vi "HorseChase.vi"() -> ()   [LabVIEW 2018]
uses:
  <vilib>/Rock Robotics/WPI/ThirdParty/Phoenix-LabVIEW/Motor Controller/Controls/CTRE_Phoenix_MotorControl_ControlMode.ctl
  <vilib>/Rock Robotics/WPI/ThirdParty/Phoenix-LabVIEW/Motor Controller/Get/CTRE_Phoenix_MotorController_GetSelectedSensorData.vi
  <vilib>/addons/control/pid/pid.llb/PID (DBL).vi
  <vilib>/addons/control/pid/NI_PID_pid.lvlib
panel:
  out "Position (Raw Sensor Units)":i32
  in  "Horse Toggle":bool
  in  "Negative":bool
  in  "Positive":bool
  in  "Boolean 7":bool
  in  "Boolean 6":bool
  in  "Numeric 2":dbl format="%#_13g"
  in  "Numeric":dbl format="%#_13g"
  in  "Boolean 5":bool
  in  "Boolean 3":bool
  in  "Boolean 4":bool
  in  "Boolean 2":bool
  in  "Boolean":bool
  in  "Max Encoder Posistion":dbl format="%#_13g"
  in  "Joystick Information":dbl format="%#_13g"
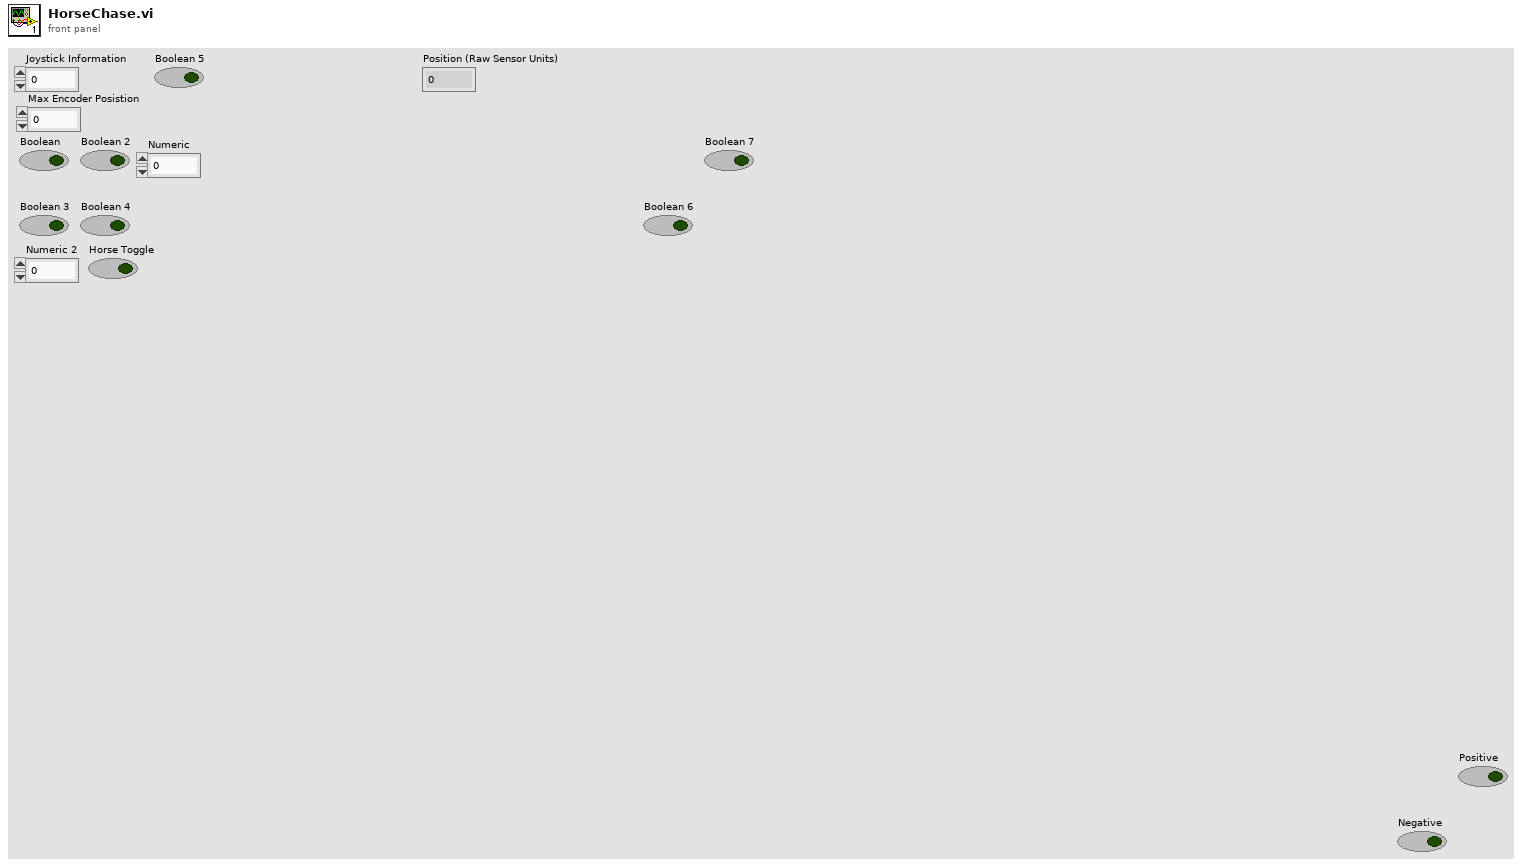
[diagram p1: front panel]
types:
  T1 = typedef "CTRE_Phoenix_MotorControl_ControlMode.ctl" = u16
  T2 = enum16{"Resting", "CargoShip Front", "CargoShip Back", "Cargo Mid", "Hatch Mid", "All High", "Cargo Intake"}
  T3 = enum16{"Resting", "Hatch Ground Intake", "Hatch Place Low/Mid/CargoShip", "Hatch Place High", "Cargo Ground Intake", "Cargo Place Low/Mid", "Cargo Place High", "CargoShip Place Front", "CargoShip Place Back"}
  T4 = cluster{"proportional gain (Kc)":dbl, "integral time (Ti, min)":dbl, "derivative time (Td, min)":dbl}
  T5 = typedef "WPI_MotorControlDeviceRef.ctl" = cluster{"DeviceStatus":errorcluster, "Type":T6, "PWM":cluster{"PWM Channel":T7, "DeadBand":T8}, "CAN":cluster{"Device Number":u8, "SetOutput VI Ref":variant, "GetOutput VI Ref":variant, "Enable VI Ref":variant, "Disable VI Ref":variant, "Data":variant}, "Invert":bool, "DIO PWM":cluster{"PWM \"Enable\" Channel":T7, "DIOChannel":T9, "PWM Rate":dbl}}
  T6 = typedef "WPI_MotorControlType.ctl" = enum16{"PWM", "CAN", "DIO PWM"}
  T7 = typedef "FPGA_DIOPWMChannel.ctl" = enum8{"PWM 0", "PWM 1", "PWM 2", "PWM 3", "PWM 4", "PWM 5", "PWM 6", "PWM 7", "PWM 8", "PWM 9", "PWM MXP 0", "PWM MXP 1", "PWM MXP 2", "PWM MXP 3", "PWM MXP 4", "PWM MXP 5", "PWM MXP 6", "PWM MXP 7", "PWM MXP 8", "PWM MXP 9", "Invalid"}
  T8 = typedef "WPI_PWMDeadband.ctl" = cluster{"Name":string, "maxPositivePwm":i32, "minPositivePwm":i32, "centerPwm":i32, "maxNegativePwm":i32, "minNegativePwm":i32, "angularRange":u16}
  T9 = typedef "FPGA_DIOChannel.ctl" = enum8{"DIO 0", "DIO 1", "DIO 2", "DIO 3", "DIO 4", "DIO 5", "DIO 6", "DIO 7", "DIO 8", "DIO 9", "DIO MXP 0", "DIO MXP 1", "DIO MXP 2", "DIO MXP 3", "DIO MXP 4", "DIO MXP 5", "DIO MXP 6", "DIO MXP 7", "DIO MXP 8", "DIO MXP 9", "DIO MXP 10", "DIO MXP 11", "DIO MXP 12", "DIO MXP 13", "DIO MXP 14", "DIO MXP 15", "SPI Port CS1", "SPI Port CS2", "SPI Port CS3", "SPI Port MISO", "SPI Port MOSI", "Invalid"}
  T10 = typedef "WPI_SwitchDevRef.ctl" = cluster{"DevStatus":errorcluster, "DIO Channel":T9, "CntIndex":T11, "Normally Closed":bool}
  T11 = typedef "FPGA_CounterCtrSystemIndex.ctl" = enum8{"Ctr 0", "Ctr 1", "Ctr 2", "Ctr 3", "Ctr 4", "Ctr 5", "Ctr 6", "Ctr 7", "Invalid"}
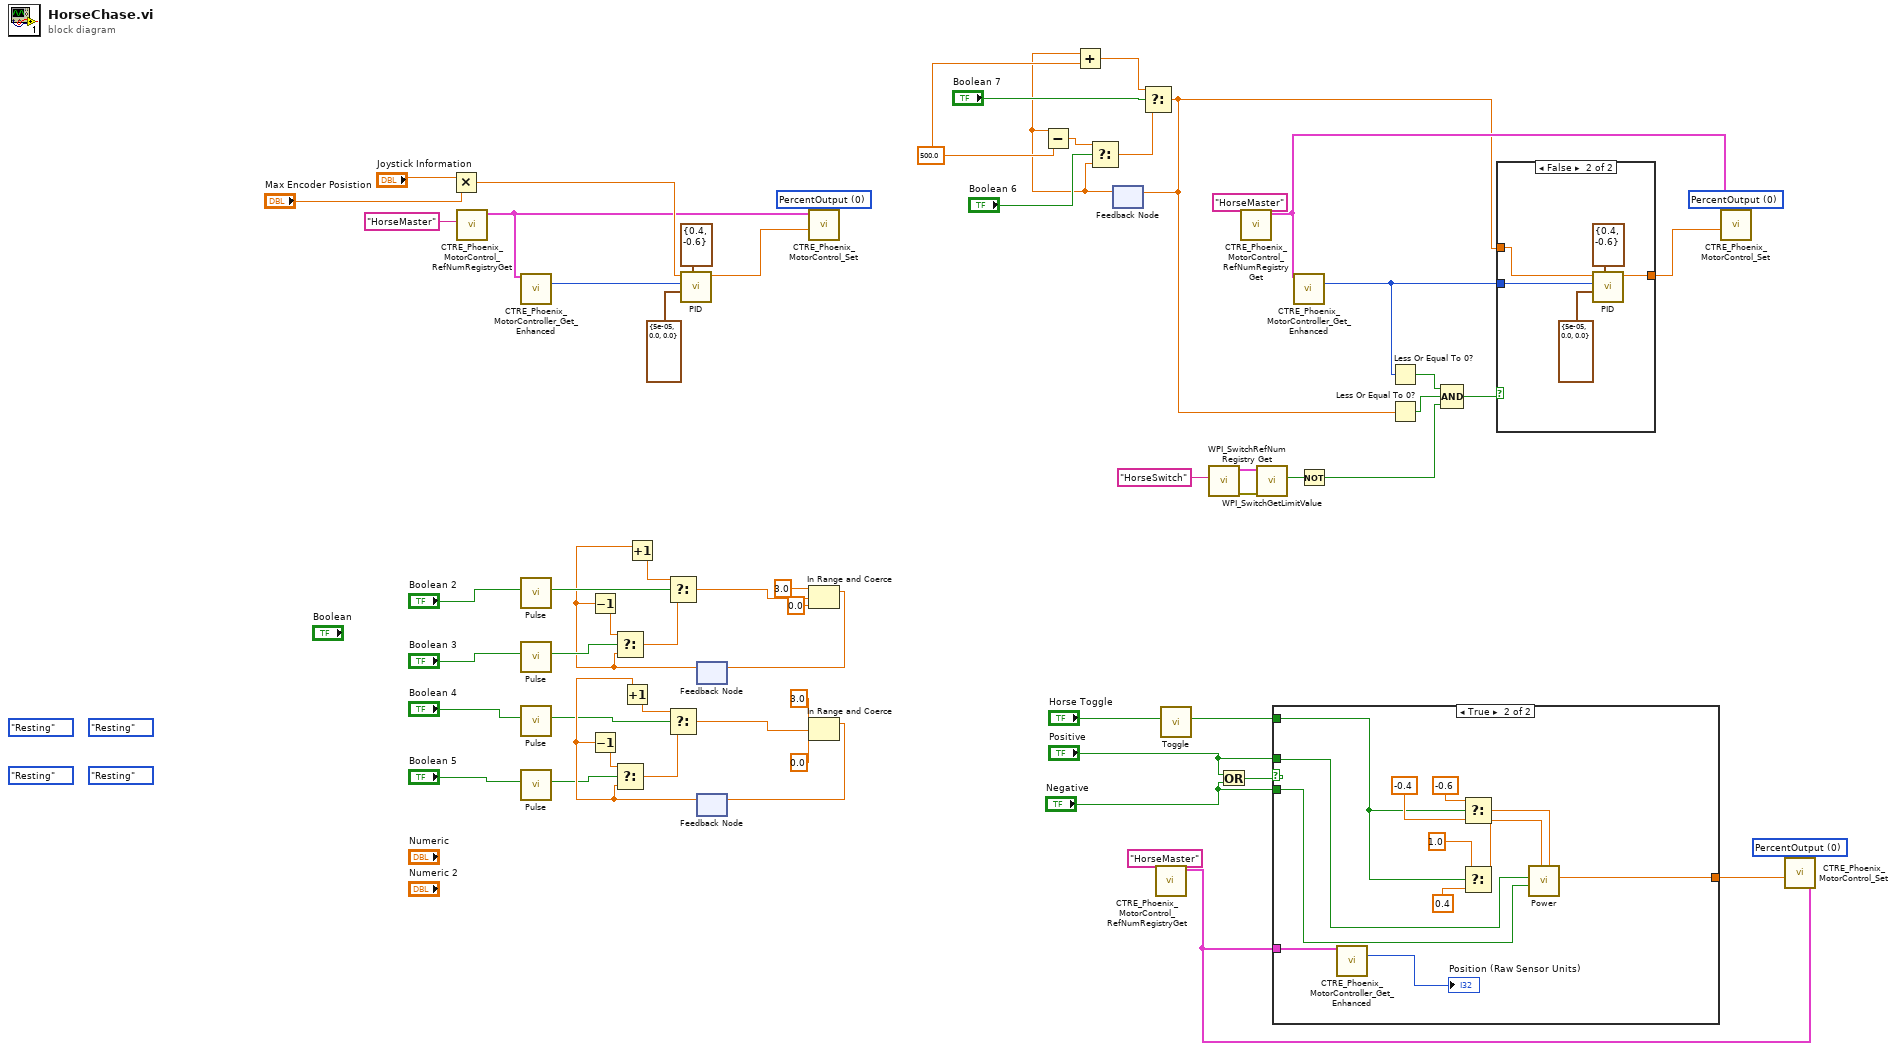
[diagram p0: block diagram]
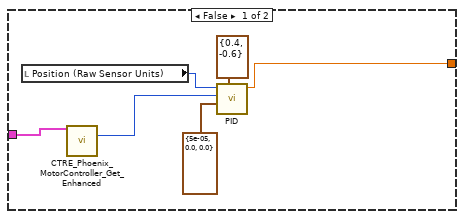
[diagram p2: hidden frame]
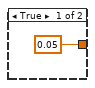
[diagram p3: hidden frame]
diagram:
  w5 = T1 0 items=["PercentOutput"=0, "Position"=1, "Velocity"=2, "Current"=3, "Follower"=5, "MotionProfile"=6, "MotionMagic"=7, "MotionProfileArc"=10, "Disabled"=15] ("Control Mode")
  (unwired) "HorseMaster" ("refnum name")
  w20 = 500.0 ("y")
  w29 = T1 0 items=["PercentOutput"=0, "Position"=1, "Velocity"=2, "Current"=3, "Follower"=5, "MotionProfile"=6, "MotionMagic"=7, "MotionProfileArc"=10, "Disabled"=15] ("Control Mode")
  (unwired) T2."Resting" ("Elevator Level Select")
  (unwired) T2."Resting" ("Elevator Level Select")
  (unwired) T3."Resting" ("Wrist")
  (unwired) T3."Resting" ("Wrist")
  w54 = T1 0 items=["PercentOutput"=0, "Position"=1, "Velocity"=2, "Current"=3, "Follower"=5, "MotionProfile"=6, "MotionMagic"=7, "MotionProfileArc"=10, "Disabled"=15] ("Control Mode")
  n1 = Multiply(x="Joystick Information", y="Max Encoder Posistion") -> (x*y=w60:dbl)
  n2 = call <vilib>:"CTRE_Phoenix_MotorControl_RefNumRegistryGet.vi"("refnum name"="HorseMaster") -> ("PhoenixMotorControlDevRef"=w55:T5)  [unwired: 9 in, 1 out]
  n3 = call-poly <vilib>:"CTRE_Phoenix_MotorController_Get_Enhanced.vi"("PhoenixMotorControlDevRef"=w55) -> ("Position (Raw Sensor Units)"=w59:i32)  [unwired: 11 in, 3 out]
  n4 = call "Pulse.vi"("Input"="Boolean 2") -> ("Output"=w52:bool)  [unwired: 10 in]
  n5 = call "Pulse.vi"("Input"="Boolean 3") -> ("Output"=w45:bool)  [unwired: 10 in]
  n6 = call "Pulse.vi"("Input"="Boolean 4") -> ("Output"=w32:bool)  [unwired: 10 in]
  n7 = call "Pulse.vi"("Input"="Boolean 5") -> ("Output"=w38:bool)  [unwired: 10 in]
  n8 = call-poly <vilib>:"PID.vi"("output range"=cluster{"output high":dbl, "output low":dbl} {"output high"=0.4, "output low"=-0.6}, "PID gains"=T4 {"proportional gain (Kc)"=5e-05, "integral time (Ti, min)"=0.0, "derivative time (Td, min)"=0.0}, "process variable"=w59, "setpoint"=w60) -> ("output"=w56:dbl)  [unwired: 6 in, 1 out]
  n9 = feedback #1() -> (w42:dbl)  [unwired: 1 in]
  n10 = Decrement(x=w42) -> (x-1=w43:dbl)
  n11 = Select(t=w43, s=w45, f=w42) -> (s? t:f=w46:dbl)
  n12 = Increment(x=w42) -> (x+1=w51:dbl)
  n13 = Select(t=w51, s=w52, f=w46) -> (s? t:f=w50:dbl)
  n14 = feedback #2() -> (w41:dbl)  [unwired: 1 in]
  n15 = Decrement(x=w41) -> (x-1=w40:dbl)
  n16 = Select(t=w40, s=w38, f=w41) -> (s? t:f=w37:dbl)
  n17 = Increment(x=w41) -> (x+1=w33:dbl)
  n18 = Select(t=w33, s=w32, f=w37) -> (s? t:f=w34:dbl)
  n19 = call <vilib>:"CTRE_Phoenix_MotorControl_Set.vi"("Output"=w56, "Control Mode"=w54, "PhoenixMotorControlDevRef"=w55) -> ()  [unwired: 7 in, 2 out]
  n20 = In Range and Coerce(upper limit=3.0, x=w50, lower limit=0.0) -> (coerced(x)=w44:dbl)  [unwired: 1 out]
  n21 = feedback-in #1(w44) -> ()
  n22 = In Range and Coerce(upper limit=3.0, x=w34, lower limit=0.0) -> (coerced(x)=w39:dbl)  [unwired: 1 out]
  n23 = feedback-in #2(w39) -> ()
  n24 = feedback #3() -> (w19:dbl)  [unwired: 1 in]
  n25 = Subtract(x=w19, y=w20) -> (x-y=w21:dbl)
  n26 = Add(x=w19, y=w20) -> (x+y=w22:dbl)
  n27 = Select(t=w21, s="Boolean 6", f=w19) -> (s? t:f=w25:dbl)
  n28 = Select(t=w22, s="Boolean 7", f=w25) -> (s? t:f=w18:dbl)
  n29 = feedback-in #3(w18) -> ()
  n30 = call <vilib>:"CTRE_Phoenix_MotorControl_RefNumRegistryGet.vi"() -> ("PhoenixMotorControlDevRef"=w4:T5)  [unwired: 10 in, 1 out]
  n31 = call "Toggle.vi"("Input"="Horse Toggle") -> ("Output"=w2:bool)  [unwired: 10 in]
  n32 = call <vilib>:"WPI_SwitchRefNum Registry Get.vi"("refnum name"="HorseSwitch") -> ("error out"=w14:errorcluster, "SwitchDevRef"=w13:T10)  [unwired: 9 in]
  n33 = Or(x="Positive", y="Negative") -> (x .or. y?=w8:bool)
  n34 = call <vilib>:"CTRE_Phoenix_MotorControl_RefNumRegistryGet.vi"("refnum name"="HorseMaster") -> ("PhoenixMotorControlDevRef"=w28:T5)  [unwired: 9 in, 1 out]
  n35 = call <vilib>:"WPI_SwitchGetLimitValue.vi"("error in (no error)"=w14, "SwitchDevRef"=w13) -> ("Switch Pressed"=w11:bool)  [unwired: 7 in, 2 out]
  n36 = case shown="True" w8 {
    tunnel: "Positive" -> [_ w75]
    tunnel: "Negative" -> [_ w74]
    tunnel: [w64 w73] -> w3
    tunnel: w4 -> [w69 w72]
    tunnel: w2 -> [_ w70]
    frame False {
      n37 = local read "Position (Raw Sensor Units)"() -> (w65:i32)
      n38 = call-poly <vilib>:"CTRE_Phoenix_MotorController_Get_Enhanced.vi"("PhoenixMotorControlDevRef"=w69) -> ("Position (Raw Sensor Units)"=w66:i32)  [unwired: 11 in, 3 out]
      n39 = call-poly <vilib>:"PID.vi"("output range"=cluster{"output high":dbl, "output low":dbl} {"output high"=0.4, "output low"=-0.6}, "PID gains"=T4 {"proportional gain (Kc)"=5e-05, "integral time (Ti, min)"=0.0, "derivative time (Td, min)"=0.0}, "process variable"=w66, "setpoint"=w65) -> ("output"=w64:dbl)  [unwired: 6 in, 1 out]
    }
    frame True {
      n40 = call-poly <vilib>:"CTRE_Phoenix_MotorController_Get_Enhanced.vi"("PhoenixMotorControlDevRef"=w72) -> ("Position (Raw Sensor Units)"=→"Position (Raw Sensor Units)":i32)  [unwired: 11 in, 3 out]
      n41 = Select(t=-0.6 ("f"), s=w70, f=-0.4) -> (s? t:f=w79:dbl)
      n42 = Select(t=1.0 ("f"), s=w70, f=0.4) -> (s? t:f=w78:dbl)
      n43 = call "Power.vi"("Negative Power"=w79, "Positive Power"=w78, "Negative"=w74, "Positive"=w75) -> ("Output"=w73:dbl)  [unwired: 7 in]
    }
  }
  n44 = call-poly <vilib>:"CTRE_Phoenix_MotorController_Get_Enhanced.vi"("PhoenixMotorControlDevRef"=w28) -> ("Position (Raw Sensor Units)"=w17:i32)  [unwired: 11 in, 3 out]
  n45 = Not(x=w11) -> (.not. x?=w10:bool)
  n46 = Less Or Equal To 0?(x=w17) -> (x <= 0?=w16:bool)
  n47 = Less Or Equal To 0?(x=w18) -> (x <= 0?=w15:bool)
  n48 = Compound Arithmetic op=AND(w16, w15, w10) -> (w9:bool)
  n49 = case shown="False" w9 {
    tunnel: [0.05 ("output") w87] -> w27
    tunnel: w17 -> [_ w84]
    tunnel: w18 -> [_ w83]
    frame True {
    }
    frame False {
      n50 = call-poly <vilib>:"PID.vi"("output range"=cluster{"output high":dbl, "output low":dbl} {"output high"=0.4, "output low"=-0.6}, "PID gains"=T4 {"proportional gain (Kc)"=5e-05, "integral time (Ti, min)"=0.0, "derivative time (Td, min)"=0.0}, "process variable"=w84, "setpoint"=w83) -> ("output"=w87:dbl)  [unwired: 6 in, 1 out]
    }
  }
  n51 = call <vilib>:"CTRE_Phoenix_MotorControl_Set.vi"("Output"=w27, "Control Mode"=w29, "PhoenixMotorControlDevRef"=w28) -> ()  [unwired: 7 in, 2 out]
  n52 = call <vilib>:"CTRE_Phoenix_MotorControl_Set.vi"("Output"=w3, "Control Mode"=w5, "PhoenixMotorControlDevRef"=w4) -> ()  [unwired: 7 in, 2 out]
